vi "TL_create_tasks_list_TDMS.vi"(4 "TL array":dbl[][](array[numeric]), 5 "error in":errorcluster, 6 "Channel #":i32, 7 "N ROIs":i32, 8 "Dt (s)":i32) -> (0 "error out":errorcluster)   [LabVIEW 2015]
uses:
  CONTROLS/Q_main_element.ctl
  GLOBAL/Global_MAIN.vi
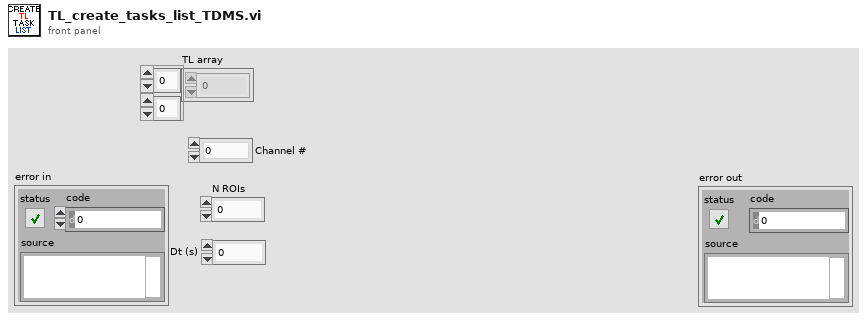
[diagram p1: front panel]
types:
  T1 = typedef "Q_main_element.ctl" = cluster{"variant":variant, "Instruction":enum16{"Main_idle", "Main_initialize", "Main_initialize_TDMS", "Main_initialize_Queue", "Main_error", "Main_DAQ_initialization_results", "Main_ASI_initialization_results", "Main_Piezo_initialization_results", "Main_Valve_initialization_results", "Main_Pump_initialization_results", "Main_CAMERA_initialization_results", "Main_DAQ_error", "Main_ASI_error", "Main_Piezo_error", "Main_CAMERA_error", "Main_Valve_error", "Main_Pump_error", "Main_start_acquiring", "Main_not_acquiring", "Main_acquiring", "Main_stop_acquiring", "Main_change_exposure", "Main_change_z_scan_parameters", "Main_define_ROI", "Main_define_mosaic", "Main_read_kinetic_time", "Main_cooler", "Main_read_temperature", "Main_save_XY", "Main_load_XY", "Main_discard_XY", "Main_move_to_XY", "Main_measure_QPD", "Main_autofocus_calibration", "Main_save_PID", "Main_change_H_valve_position", "Main_two_way_valve", "Main_save_movie", "Main_init_single_scan", "Main_single_scan", "Main_stop_single_scan", "Main_merFISH_illumination_parameters", "Main_merFISH_buffer_probe_list", "Main_merFISH_injections_procedure", "Main_merFISH_save_setpoint", "Main_merFISH_DAPI_parameters", "Main_merFISH_Brightfield_parameters", "Main_merFISH_save_embryo_ROI", "Main_merFISH_init", "Main_merFISH_resume", "Main_merFISH_start_autofocus", "Main_merFISH_open_close_valve_merFISH", "Main_merFISH_open_close_valve_photobleaching", "Main_merFISH_hybridization", "Main_merFISH_move_to_ROI", "Main_merFISH_wait_stabilization", "Main_merFISH_scan_laser", "Main_merFISH_scan_brightfield", "Main_merFISH_photobleaching_injection", "Main_merFISH_photobleaching", "Main_merFISH_save", "Main_merFISH_send_email", "Main_merFISH_close", "Main_TL_define_parameters", "Main_TL_reset_parameters", "Main_TL_init", "Main_TL_start_autofocus", "Main_TL_move_to_ROI", "Main_TL_wait_for_stabilization", "Main_TL_scan", "Main_TL_wait_cycle_end", "Main_TL_close", "Main_STOP"}}
  T2 = enum16{"open", "open or create", "create or replace", "create", "open (read-only)"}
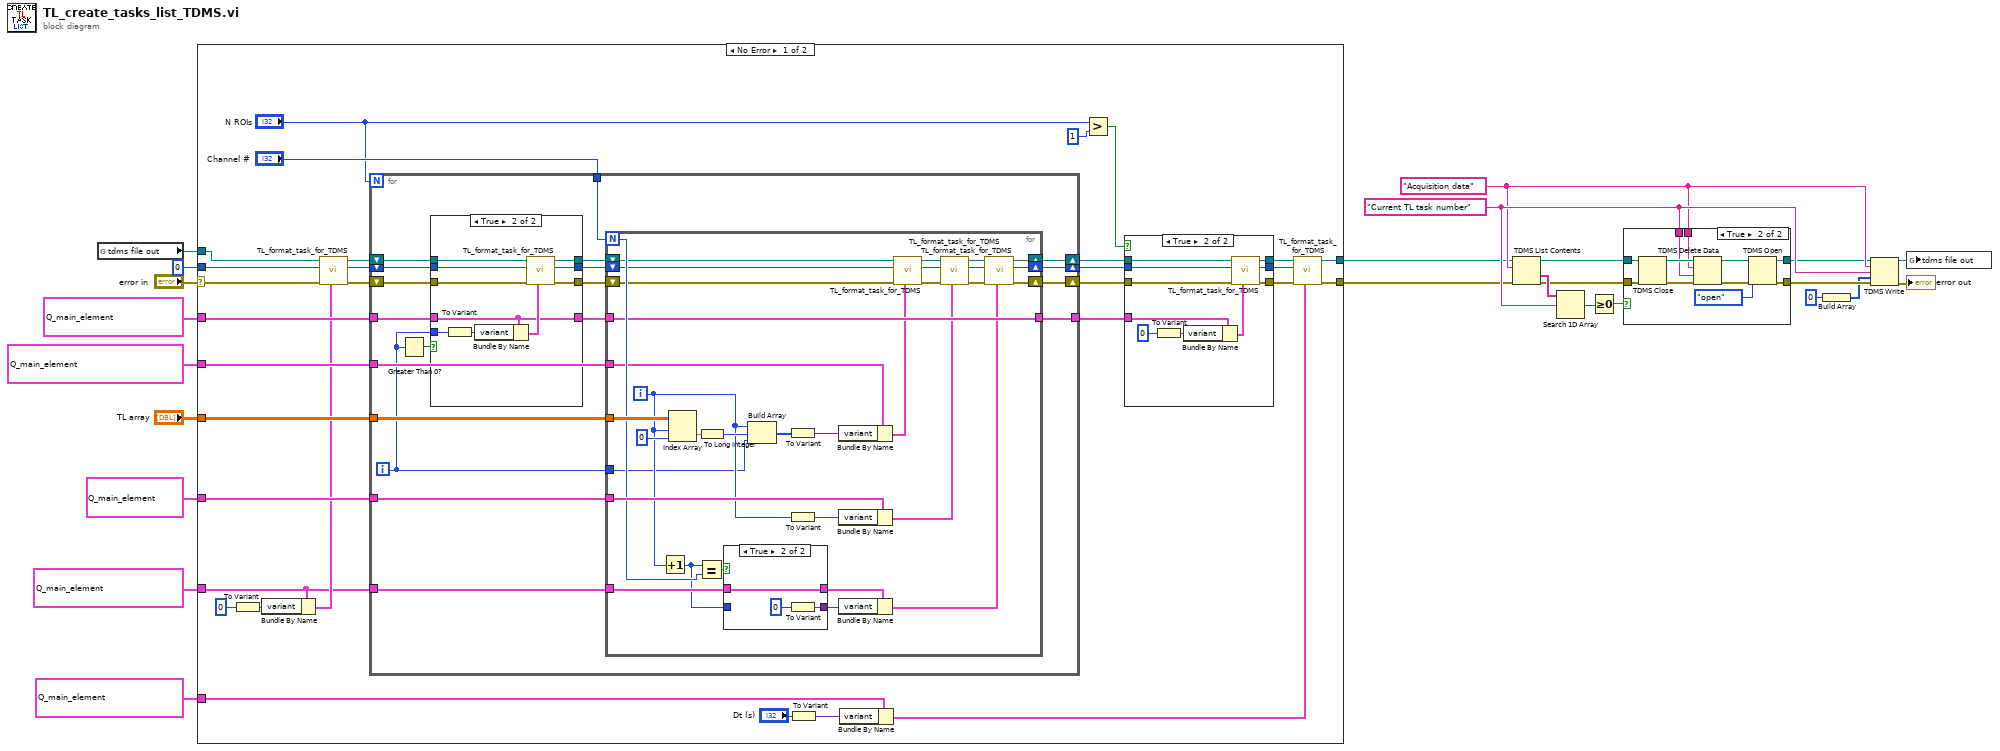
[diagram p0: block diagram]
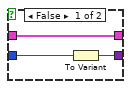
[diagram p5: hidden frame]
diagram:
  w12 = "Current TL task number" ("group name in")
  w11 = "Acquisition data" ("group name in")
  n1 = global read "Global_MAIN.vi" "tdms file out"() -> (w16:refnum<k34>)
  n2 = case shown="No Error" "error in" {
    selector: "error in" -> [w41 w142]
    tunnel: T1 {"variant"=variant, "Instruction"=enum."Main_TL_wait_for_stabilization"} ("element") -> [w55 _]
    tunnel: T1 {"variant"=variant, "Instruction"=enum."Main_TL_scan"} ("element") -> [w54 _]
    tunnel: T1 {"variant"=variant, "Instruction"=enum."Main_TL_move_to_ROI"} ("element") -> [w51 _]
    tunnel: T1 {"variant"=variant, "Instruction"=enum."Main_TL_wait_cycle_end"} ("element") -> [w53 _]
    tunnel: "TL array" -> [w46 _]
    tunnel: T1 {"variant"=variant, "Instruction"=enum."Main_TL_start_autofocus"} ("element") -> [w25 _]
    tunnel: 0 ("index (row)") -> [w39 _]
    tunnel: w16 -> [w38 w141]
    tunnel: [w27 w142] -> w2
    tunnel: [w26 w141] -> w3
    frame No Error {
      n3 = To Variant(anything=0 ("index (row)")) -> (Variant=w50:variant)
      n4 = Bundle By Name(cluster=w25, "variant"=w50) -> (w40:T1)
      n5 = call "TL_format_task_for_TDMS.vi"("Task"=w40, "error in"=w41, "Task number"=w39, "tdms file"=w38) -> ("error out"=w37:errorcluster, "Next task number"=w36:i32, "tdms file out"=w35:refnum<k34>)  [unwired: 2 in]
      n6 = for {
        N: "N ROIs" -> [_]
        tunnel: w55 -> [w86]
        tunnel: w54 -> [w85]
        tunnel: w51 -> [w81]
        tunnel: "Channel #" -> [w87]
        tunnel: w46 -> [w84]
        tunnel: w25 -> [w83]
        tunnel: [w82] -> w45
        shift-right: [w70] -> w33
        shift-left: w36 -> [w77]
        shift-right: [w71] -> w34
        shift-left: w35 -> [w78]
        shift-right: [w69] -> w32
        shift-left: w37 -> [w76]
        i -> [w79]
        n7 = Greater Than 0?(x=w79) -> (x > 0?=w80:bool)
        n8 = case shown="True" w80 {
          tunnel: w79 -> [_ w100]
          tunnel: w81 -> [w88 w92]
          tunnel: w78 -> [w91 w99]
          tunnel: w77 -> [w90 w98]
          tunnel: w76 -> [w89 w97]
          tunnel: [w89 w95] -> w73
          tunnel: [w90 w94] -> w74
          tunnel: [w91 w93] -> w75
          tunnel: [w88 w92] -> w72
          frame False {
          }
          frame True {
            n9 = To Variant(anything=w100) -> (Variant=w101:variant)
            n10 = Bundle By Name(cluster=w92, "variant"=w101) -> (w96:T1)
            n11 = call "TL_format_task_for_TDMS.vi"("Task"=w96, "error in"=w97, "Task number"=w98, "tdms file"=w99) -> ("error out"=w95:errorcluster, "Next task number"=w94:i32, "tdms file out"=w93:refnum<k34>)  [unwired: 2 in]
          }
        }
        n12 = for {
          N: w87 -> [w124]
          tunnel: w86 -> [w122]
          tunnel: w85 -> [w129]
          tunnel: w84 -> [w134]
          tunnel: w79 -> [w118]
          tunnel: w83 -> [w127]
          tunnel: [w121] -> w82
          tunnel: w72 -> [w121]
          shift-right: [w102] -> w71
          shift-left: w75 -> [w116]
          shift-right: [w103] -> w70
          shift-left: w74 -> [w115]
          shift-right: [w104] -> w69
          shift-left: w73 -> [w114]
          i -> [w119]
          n13 = Increment(x=w119) -> (x+1=w123:i32)
          n14 = Index Array(array=w134, index (row)=w119, index (col)=0 ("disabled index (col)")) -> (element=w132:dbl)
          n15 = To Long Integer(number=w132) -> (32bit integer=w120:i32)
          n16 = Equal?(x=w123, y=w124) -> (x = y?=w128:bool)
          n17 = case shown="True" w128 {
            tunnel: w127 -> [w137 w140]
            tunnel: [w137 w140] -> w126
            tunnel: [w136 w139] -> w125
            tunnel: w123 -> [w135 _]
            frame False {
              n18 = To Variant(anything=w135) -> (Variant=w136:variant)
            }
            frame True {
              n19 = To Variant(anything=0 ("disabled index (col)")) -> (Variant=w139:variant)
            }
          }
          n20 = Build Array(w119, w120, w118) -> (w117:i32[])
          n21 = To Variant(anything=w117) -> (Variant=w131:variant)
          n22 = To Variant(anything=w119) -> (Variant=w130:variant)
          n23 = Bundle By Name(cluster=w122, "variant"=w131) -> (w113:T1)
          n24 = Bundle By Name(cluster=w129, "variant"=w130) -> (w109:T1)
          n25 = Bundle By Name(cluster=w126, "variant"=w125) -> (w105:T1)
          n26 = call "TL_format_task_for_TDMS.vi"("Task"=w113, "error in"=w114, "Task number"=w115, "tdms file"=w116) -> ("error out"=w110:errorcluster, "Next task number"=w111:i32, "tdms file out"=w112:refnum<k34>)  [unwired: 2 in]
          n27 = call "TL_format_task_for_TDMS.vi"("Task"=w109, "error in"=w110, "Task number"=w111, "tdms file"=w112) -> ("error out"=w108:errorcluster, "Next task number"=w107:i32, "tdms file out"=w106:refnum<k34>)  [unwired: 2 in]
          n28 = call "TL_format_task_for_TDMS.vi"("Task"=w105, "error in"=w108, "Task number"=w107, "tdms file"=w106) -> ("error out"=w104:errorcluster, "Next task number"=w103:i32, "tdms file out"=w102:refnum<k34>)  [unwired: 2 in]
        }
      }
      n29 = To Variant(anything="Dt (s)") -> (Variant=w52:variant)
      n30 = Bundle By Name(cluster=w53, "variant"=w52) -> (w28:T1)
      n31 = Greater?(x="N ROIs", y=1) -> (0:w42:bool)
      n32 = case shown="True" w42 {
        tunnel: w45 -> [_ w67]
        tunnel: [w58 w65] -> w29
        tunnel: w34 -> [w56 w64]
        tunnel: w33 -> [w57 w63]
        tunnel: w32 -> [w58 w62]
        tunnel: [w57 w59] -> w30
        tunnel: [w56 w60] -> w31
        frame False {
        }
        frame True {
          n33 = To Variant(anything=0 ("index (row)")) -> (Variant=w68:variant)
          n34 = Bundle By Name(cluster=w67, "variant"=w68) -> (w61:T1)
          n35 = call "TL_format_task_for_TDMS.vi"("Task"=w61, "error in"=w62, "Task number"=w63, "tdms file"=w64) -> ("error out"=w65:errorcluster, "Next task number"=w59:i32, "tdms file out"=w60:refnum<k34>)  [unwired: 2 in]
        }
      }
      n36 = call "TL_format_task_for_TDMS.vi"("Task"=w28, "error in"=w29, "Task number"=w30, "tdms file"=w31) -> ("error out"=w27:errorcluster, "tdms file out"=w26:refnum<k34>)  [unwired: 2 in, 1 out]
    }
    frame Error {
    }
  }
  n37 = TDMS List Contents(4:w2, 6:w11, 7:w3) -> (0:w5:errorcluster, 1:w8:string[], 3:w6:refnum<k34>)  [unwired: 1 out]
  n38 = Search 1D Array(1D array=w8, element=w12) -> (index of element=w7:i32)  [unwired: 1 in]
  n39 = Greater Or Equal To 0?(x=w7) -> (x >= 0?=w4:bool)
  n40 = case shown="True" w4 {
    tunnel: [w144 w152] -> w9
    tunnel: [w143 w151] -> w14
    tunnel: w6 -> [w144 w148]
    tunnel: w5 -> [w143 w147]
    tunnel: w12 -> [_ w146]
    tunnel: w11 -> [_ w145]
    frame False {
    }
    frame True {
      n41 = TDMS Close(8:w147, 11:w148) -> (0:w149:errorcluster, 3:w150:path)
      n42 = TDMS Delete Data(8:w149, 9:w146, 10:w145, 11:w150) -> (0:w154:errorcluster, 3:w155:path)  [unwired: 3 in]
      n43 = TDMS Open(8:w154, 10:T2."open" ("operation (0:open)"), 11:w155) -> (0:w151:errorcluster, 3:w152:refnum<k34>)  [unwired: 4 in]
    }
  }
  n44 = Build Array(u32 0) -> (w10:u32[])
  n45 = TDMS Write(0:w9, 5:w11, 7:w12, 9:w10, 11:w14) -> (4:w13:refnum<k34>, 15:→"error out":errorcluster)  [unwired: 1 in, 2 out]
  n46 = global write "Global_MAIN.vi" "tdms file out"(w13) -> ()
